vi "Min-Max Defaults.vi"(8 "error in (no error)":errorcluster, 11 "Numeric Data Type in":refnum<class "Numeric Data Type.lvclass">) -> (0 "error out":errorcluster, 1 "Maximum":dbl, 2 "Minimum":dbl, 3 "Numeric Data Type (dup)":refnum<class "Numeric Data Type.lvclass">, 4 "Increment":dbl)   [LabVIEW 2018, in "Numeric Data Type.lvclass"]
uses:
  Numeric Data Type.lvclass
  Numeric Data Type.lvclass/Numeric Data Type.ctl
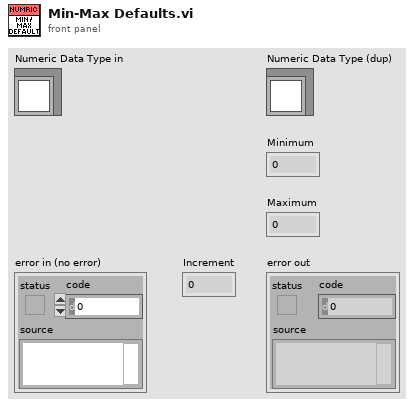
[diagram p1: front panel]
types:
  T1 = typedef "Numeric Data Type.lvclass/Representation Enum.ctl" = enum16{"Extended (EXT)", "Double (DBL)", "Single (SGL)", "Fixed-Point (FXP)", "Quad Integer (I64)", "Long Integer (I32)", "Word Integer (I16)", "Byte Integer (I8)", "Unsigned Quad (U64)", "Unsigned Long (U32)", "Unsigned Word (U16)", "Unsigned Byte (U8)", "Complex Extended (CXT)", "Complex Double (CDB)", "Complex Single (CSG)"}
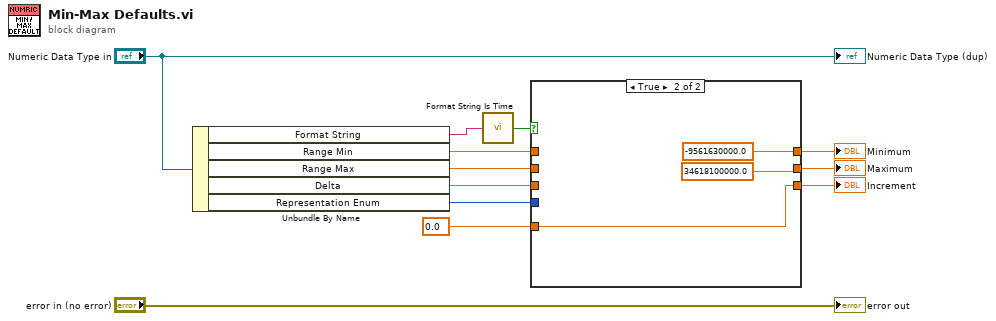
[diagram p0: block diagram]
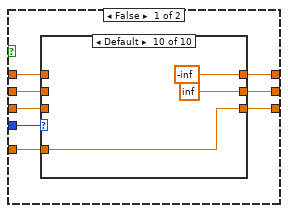
[diagram p2: hidden frame]
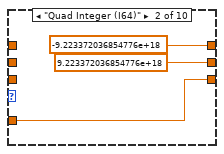
[diagram p4: hidden frame]
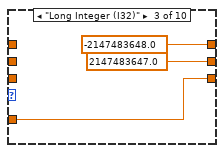
[diagram p5: hidden frame]
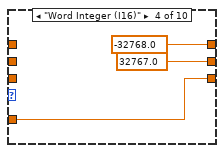
[diagram p6: hidden frame]
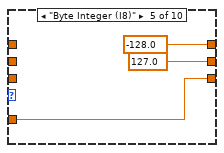
[diagram p7: hidden frame]
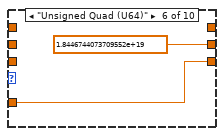
[diagram p8: hidden frame]
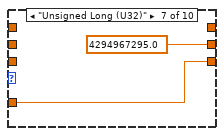
[diagram p9: hidden frame]
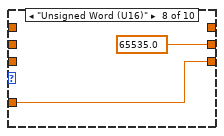
[diagram p10: hidden frame]
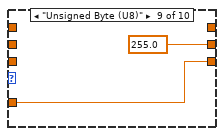
[diagram p11: hidden frame]
diagram:
  n1 = Unbundle By Name("Numeric Data Type in") -> ("Format String"=w2:string, "Range Min"=w5:dbl, "Range Max"=w6:dbl, "Delta"=w7:dbl, "Representation Enum"=w8:T1)
  n2 = call "Format String Is Time.vi"("Format String"=w2) -> ("Time?"=w1:bool)
  n3 = case shown="True" w1 {
    tunnel: [w20 -9561630000.0 ("Range Min")] -> w11
    tunnel: [w19 34618100000.0 ("Range Max")] -> w10
    tunnel: [w18 w47] -> w9
    tunnel: w8 -> [w17 _]
    tunnel: w7 -> [w16 _]
    tunnel: w6 -> [w15 _]
    tunnel: w5 -> [w14 _]
    tunnel: 0.0 -> [w13 w47]
    frame False {
      n4 = case shown="Default" w17 {
        tunnel: [w22 9.223372036854776e+18 2147483647.0 32767.0 127.0 1.8446744073709552e+19 4294967295.0 65535.0 255.0 inf] -> w19
        tunnel: [w23 -9.223372036854776e+18 -2147483648.0 -32768.0 -128.0 _ _ _ _ -inf] -> w20
        tunnel: w16 -> [w21 _ _ _ _ _ _ _ _ _]
        tunnel: w15 -> [w22 _ _ _ _ _ _ _ _ _]
        tunnel: w14 -> [w23 _ _ _ _ _ _ _ _ _]
        tunnel: [w21 w24 w27 w30 w33 w36 w38 w40 w42 w44] -> w18
        tunnel: w13 -> [_ w24 w27 w30 w33 w36 w38 w40 w42 w44]
        frame "Fixed-Point (FXP)" {
        }
        frame "Quad Integer (I64)" {
        }
        frame "Long Integer (I32)" {
        }
        frame "Word Integer (I16)" {
        }
        frame "Byte Integer (I8)" {
        }
        frame "Unsigned Quad (U64)" {
        }
        frame "Unsigned Long (U32)" {
        }
        frame "Unsigned Word (U16)" {
        }
        frame "Unsigned Byte (U8)" {
        }
        frame Default {
        }
      }
    }
    frame True {
    }
  }
  "Minimum" <- w11
  "Maximum" <- w10
  "Increment" <- w9
  "error out" <- "error in (no error)"
  "Numeric Data Type (dup)" <- "Numeric Data Type in"
